vi "Drive PID.vi"(11 "Setpoint":dbl) -> (3 "Done":bool)   [LabVIEW 2015]
uses:
  <vilib>/Rock Robotics/Network Tables/NT Read Number.vi
  <vilib>/Rock Robotics/WPI/Utilities/WPI_GetSetVariantRefNum.vi
  <vilib>/addons/control/pid/pid.llb/PID (DBL).vi
  <vilib>/addons/control/pid/NI_PID_pid.lvlib
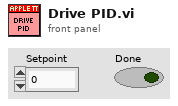
[diagram p1: front panel]
types:
  T1 = typedef "WPI_EncoderDevRef.ctl" = cluster{"DevStatus":errorcluster, "EncoderIndex":T2, "CounterIndex":T3, "DistancePerCount":dbl, "Decoding Type":T4}
  T2 = typedef "FPGA_EncoderIdx.ctl" = enum8{"Enc 0", "Enc 1", "Enc 2", "Enc 3", "Enc 4", "Enc 5", "Enc 6", "Enc 7", "Invalid"}
  T3 = typedef "FPGA_CounterCtrSystemIndex.ctl" = enum8{"Ctr 0", "Ctr 1", "Ctr 2", "Ctr 3", "Ctr 4", "Ctr 5", "Ctr 6", "Ctr 7", "Invalid"}
  T4 = typedef "WPI_EncoderType.ctl" = enum16{"1x", "2x", "4x"}
  T5 = cluster{"proportional gain (Kc)":dbl, "integral time (Ti, min)":dbl, "derivative time (Td, min)":dbl}
  T6 = typedef "WPI_RobotDriveDevRef.ctl" = cluster{"DevStatus":errorcluster, "Motors[]":T7[], "Square Inputs":bool, "Max Output":dbl}
  T7 = typedef "WPI_MotorControlDeviceRef.ctl" = cluster{"DeviceStatus":errorcluster, "Type":T8, "PWM":cluster{"PWM Channel":T9, "DeadBand":T10}, "CAN":cluster{"Device Number":u8, "Control Mode":T11, "Semaphore":T12, "Max Vout":dbl, "TalonSRX Control Mode":T13}, "Invert":bool}
  T8 = typedef "WPI_MotorControlType.ctl" = enum16{"PWM", "CAN", "CANTalonSRX"}
  T9 = typedef "FPGA_DIOPWMChannel.ctl" = enum8{"PWM 0", "PWM 1", "PWM 2", "PWM 3", "PWM 4", "PWM 5", "PWM 6", "PWM 7", "PWM 8", "PWM 9", "PWM MXP 0", "PWM MXP 1", "PWM MXP 2", "PWM MXP 3", "PWM MXP 4", "PWM MXP 5", "PWM MXP 6", "PWM MXP 7", "PWM MXP 8", "PWM MXP 9", "Invalid"}
  T10 = typedef "WPI_PWMDeadband.ctl" = cluster{"Name":string, "maxPositivePwm":i32, "minPositivePwm":i32, "centerPwm":i32, "maxNegativePwm":i32, "minNegativePwm":i32, "angularRange":u16}
  T11 = typedef "WPI_CANJaguar_ControlMode.ctl" = enum8{"Percent VBus", "Current", "Speed", "Position", "Voltage"}
  T12 = typedef "Semaphore RefNum" = refnum<k1>
  T13 = typedef "WPI_CANTalonSRX_APIControlMode.ctl" = enum8{"Percent VBus", "Speed", "Position", "Slave", "Unchanged / Invalid", "Voltage Compensation", "Current", "Motion Profile"}
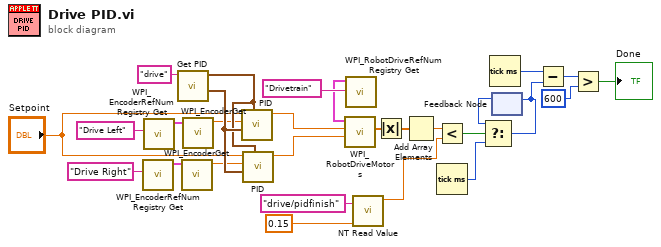
[diagram p0: block diagram]
diagram:
  n1 = call <vilib>:"WPI_EncoderRefNum Registry Get.vi"("refnum name"="Drive Right") -> ("EncoderDevRef"=w28:T1)  [unwired: 9 in, 1 out]
  n2 = call <vilib>:"WPI_EncoderRefNum Registry Get.vi"("refnum name"="Drive Left") -> ("EncoderDevRef"=w27:T1)  [unwired: 9 in, 1 out]
  n3 = call "Get PID.vi"("Subsystem"="drive") -> ("PID Gains"=w13:T5, "output range"=w12:cluster{"output high":dbl, "output low":dbl})  [unwired: 8 in]
  n4 = call <vilib>:"WPI_EncoderGet.vi"("EncoderDevRef"=w28) -> ("Distance"=w7:dbl)  [unwired: 5 in, 5 out]
  n5 = call <vilib>:"WPI_EncoderGet.vi"("EncoderDevRef"=w27) -> ("Distance"=w6:dbl)  [unwired: 5 in, 5 out]
  n6 = call-poly <vilib>:"PID.vi"("output range"=w12, "PID gains"=w13, "process variable"=w6, "setpoint"="Setpoint") -> ("output"=w9:dbl)  [unwired: 6 in, 1 out]
  n7 = call-poly <vilib>:"PID.vi"("output range"=w12, "PID gains"=w13, "process variable"=w7, "setpoint"="Setpoint") -> ("output"=w10:dbl)  [unwired: 6 in, 1 out]
  n8 = call <vilib>:"WPI_RobotDriveRefNum Registry Get.vi"("refnum name"="Drivetrain") -> ("RobotDriveDevRef"=w4:T6)  [unwired: 9 in, 1 out]
  n9 = call <vilib>:"WPI_RobotDriveMotors.vi"("RightSpeed"=w10, "LeftSpeed"=w9, "RobotDriveDevRef"=w4) -> ("Motor Values"=w14:dbl[])  [unwired: 6 in, 2 out]
  n10 = call-poly <vilib>:"NT Read Value.vi"("Default Value"=0.15, "Name"="drive/pidfinish") -> ("Numeric"=w2:dbl)  [unwired: 8 in, 1 out]
  n11 = Absolute Value(x=w14) -> (abs(x)=w15:dbl[])
  n12 = Add Array Elements(numeric array=w15) -> (sum=w16:dbl)
  n13 = Less?(x=w16, y=w2) -> (x < y?=w17:bool)
  n14 = Tick Count (ms)() -> (millisecond timer value=w18:u32)
  n15 = Tick Count (ms)() -> (millisecond timer value=w20:u32)
  n16 = feedback #1() -> (w19:u32)  [unwired: 1 in]
  n17 = Select(t=w19, s=w17, f=w18) -> (s? t:f=w21:u32)
  n18 = feedback-in #1(w21) -> ()
  n19 = Subtract(x=w20, y=w21) -> (x-y=w22:u32)
  n20 = Greater?(x=w22, y=u32 600) -> (0:→"Done":bool)
